vi "AlliGator Refnums Storage.vi"(6 "Get(F)/Set":bool, 7 "AlliGator Refnum List":T1, 8 "Error In":errorcluster, 11 "Data in":variant) -> (0 "Error Out":errorcluster, 3 "Data out":variant)   [LabVIEW 2021, in "AlliGator Globals, Variables & Constants.lvlib"]
doc: "LV2-type global storing refnums to VIs, Tabs and Indicators."
uses:
  AlliGator Globals, Variables & Constants.lvlib
  AlliGator Refnums List.ctl
  GUI/AlliGator Main Window Tabs.ctl
  GUI/AlliGator GUI.lvlib
panel:
  in  "Tab Control":enum32{"Controls", "Indicators", "VIs"}(tab)
  in  "AlliGator Tab Control Refnum":refnum<vi>
  in  "Phasor Plot Display":refnum<vi>
  in  "Decay Fit Parameter Map Display":refnum<vi> caption="Source Image Display"
  in  "Source Image Display":refnum<vi>
  in  "AlliGator Launcher  Refnum":refnum<vi>
  in  "AlliGator Settings Refnum":refnum<vi>
  in  "AlliGator Refnum":refnum<vi>
  # "see the AlliGator License on the block diagram (Ctrl+E or Window:Show Block Diagram)"
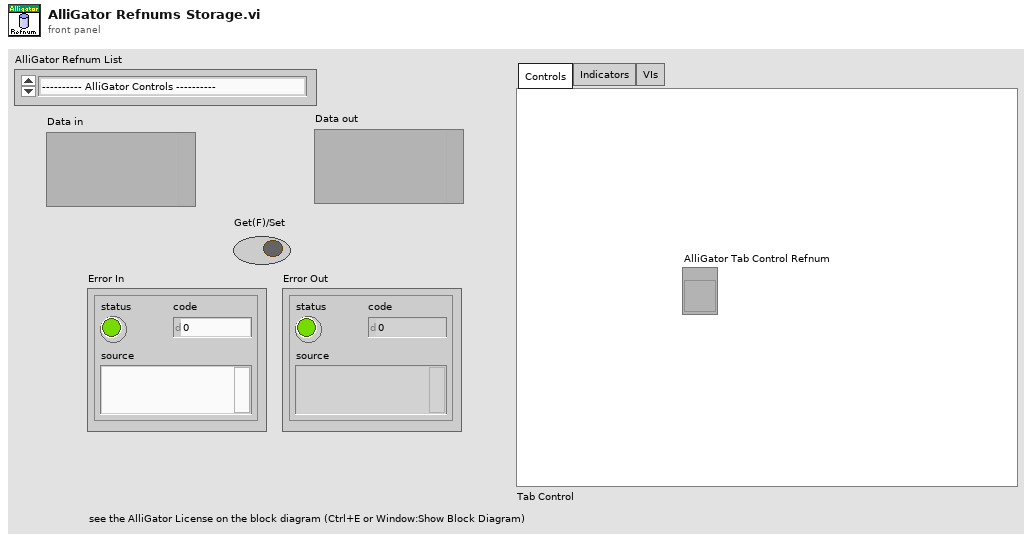
[diagram p1: front panel]
types:
  T1 = typedef "AlliGator Globals, Variables & Constants.lvlib/AlliGator Refnums List.ctl" = enum16{"---------- AlliGator Controls ----------", "AlliGator Tab Control Refnum", "---------- AlliGator Indicators ----------", "Source Image Display Refnum", "Phasor Plot Display Refnum", "Decay Fit Parameter Map Refnum", "---------- AlliGator VIs ----------", "AlliGator Refnum", "AlliGator Settings Refnum", "AlliGator Launcher Refnum"}
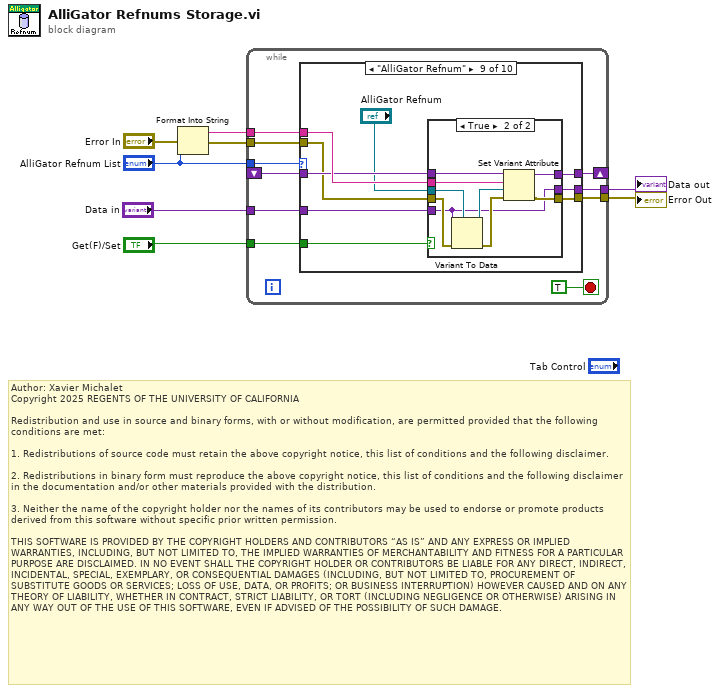
[diagram p0: block diagram]
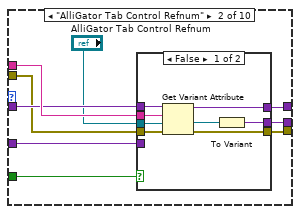
[diagram p3: hidden frame]
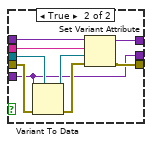
[diagram p4: hidden frame]
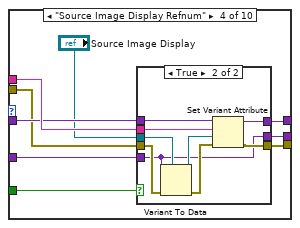
[diagram p6: hidden frame]
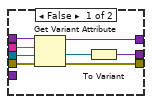
[diagram p7: hidden frame]
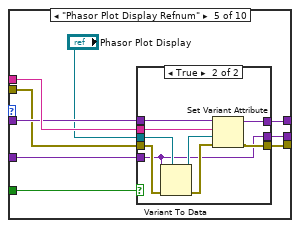
[diagram p8: hidden frame]
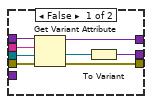
[diagram p9: hidden frame]
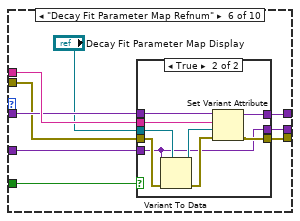
[diagram p10: hidden frame]
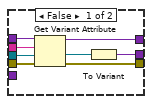
[diagram p11: hidden frame]
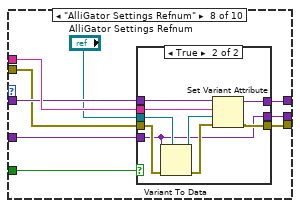
[diagram p13: hidden frame]
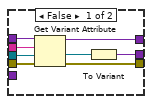
[diagram p14: hidden frame]
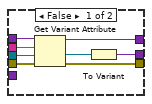
[diagram p15: hidden frame]
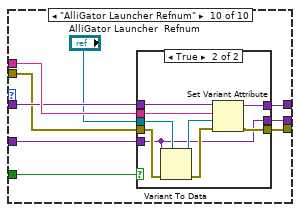
[diagram p16: hidden frame]
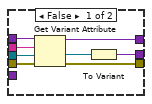
[diagram p17: hidden frame]
diagram:
  # "Author: Xavier Michalet\nCopyright 2025 REGENTS OF THE UNIVERSITY OF CALIFORNIA\n\nRedistribution and use in source and binary forms, with or without modification, are permitted provided that the following conditions are met:\n\n1. Redistributions of source code must retain the above copyright notice, this list of conditions and the following disclaimer.\n\n2. Redistributions in binary form must reproduce the above copyright notice, this list of conditions and the following disclaimer in the documentation and/or other materials provided with the distribution.\n\n3. Neither the name of the copyright holder nor the names of its contributors may be used to endorse or promote products derived from this software without specific prior written permission.\n\nTHIS SOFTWARE IS PROVIDED BY THE COPYRIGHT HOLDERS AND CONTRIBUTORS “AS IS” AND ANY EXPRESS OR IMPLIED WARRANTIES, INCLUDING, BUT NOT LIMITED TO, THE IMPLIED WARRANTIES OF MERCHANTABILITY AND FITNESS FOR A PARTICULAR PURPOSE ARE DISCLAIMED. IN NO EVENT SHALL THE COPYRIGHT HOLDER OR CONTRIBUTORS BE LIABLE FOR ANY DIRECT, INDIRECT, INCIDENTAL, SPECIAL, EXEMPLARY, OR CONSEQUENTIAL DAMAGES (INCLUDING, BUT NOT LIMITED TO, PROCUREMENT OF SUBSTITUTE GOODS OR SERVICES; LOSS OF USE, DATA, OR PROFITS; OR BUSINESS INTERRUPTION) HOWEVER CAUSED AND ON ANY THEORY OF LIABILITY, WHETHER IN CONTRACT, STRICT LIABILITY, OR TORT (INCLUDING NEGLIGENCE OR OTHERWISE) ARISING IN ANY WAY OUT OF THE USE OF THIS SOFTWARE, EVEN IF ADVISED OF THE POSSIBILITY OF SUCH DAMAGE."
  n1 = Format Into String(error in="Error In", "AlliGator Refnum List") -> (resulting string=w7:string, error out=w4:errorcluster)  [unwired: 2 in]
  n2 = while {
    tunnel: "Get(F)/Set" -> [w11]
    tunnel: w7 -> [w17]
    shift-right: [w15] -> _
    shift-left: _ -> [w16]
    tunnel: "Data in" -> [w10]
    tunnel: w4 -> [w14]
    tunnel: [w13] -> w3
    tunnel: [w12] -> w2
    tunnel: "AlliGator Refnum List" -> [w9]
    stop <- TRUE stop-if-true
    n3 = case shown="\"AlliGator Refnum\"" w9 {
      tunnel: w17 -> [_ w30 _ w59 w85 w111 _ w140 w166 w192]
      tunnel: w16 -> [w20 w29 w50 w58 w84 w110 w130 w139 w165 w191]
      tunnel: [w20 w28 w50 w57 w83 w109 w130 w138 w164 w190] -> w15
      tunnel: w14 -> [w21 w27 w48 w56 w82 w108 w131 w137 w163 w189]
      tunnel: [w21 w26 w48 w55 w81 w107 w131 w136 w162 w188] -> w13
      tunnel: [w19 w25 w49 w54 w80 w106 w129 w135 w161 w187] -> w12
      tunnel: w11 -> [_ w24 _ w53 w79 w105 _ w134 w160 w186]
      tunnel: w10 -> [w19 w23 w49 w52 w78 w104 w129 w133 w159 w185]
      frame "---------- AlliGator Controls ----------", Default {
      }
      frame "AlliGator Tab Control Refnum" {
        n4 = case shown="False" w24 {
          tunnel: w29 -> [w38 w47]
          tunnel: w30 -> [w37 w42]
          tunnel: w27 -> [w36 w46]
          tunnel: [w35 w40] -> w26
          tunnel: [w31 w39] -> w25
          tunnel: [w33 w41] -> w28
          tunnel: "AlliGator Tab Control Refnum" -> [w32 w45]
          tunnel: w23 -> [_ w39]
          frame False {
            n5 = Get Variant Attribute(Variant=w38, name=w37, default value (empty Variant)=w32, error in=w36) -> (duplicate Variant=w33:variant, value=w34:refnum<vi>, error out=w35:errorcluster)  [unwired: 1 out]
            n6 = To Variant(anything=w34) -> (Variant=w31:variant)
          }
          frame True {
            n7 = Variant To Data(error in=w46, type=w45, Variant=w39) -> (data=w44:refnum<vi>, error out=w43:errorcluster)
            n8 = Set Variant Attribute(Variant=w47, name=w42, value=w44, error in=w43) -> (Variant out=w41:variant, error out=w40:errorcluster)  [unwired: 1 out]
          }
        }
      }
      frame "---------- AlliGator Indicators ----------" {
      }
      frame "Source Image Display Refnum" {
        n9 = case shown="True" w53 {
          tunnel: w58 -> [w67 w76]
          tunnel: w59 -> [w66 w71]
          tunnel: w56 -> [w65 w75]
          tunnel: [w64 w69] -> w55
          tunnel: [w60 w68] -> w54
          tunnel: [w62 w70] -> w57
          tunnel: "Source Image Display" -> [w61 w74]
          tunnel: w52 -> [_ w68]
          frame False {
            n10 = Get Variant Attribute(Variant=w67, name=w66, default value (empty Variant)=w61, error in=w65) -> (duplicate Variant=w62:variant, value=w63:refnum<vi>, error out=w64:errorcluster)  [unwired: 1 out]
            n11 = To Variant(anything=w63) -> (Variant=w60:variant)
          }
          frame True {
            n12 = Variant To Data(error in=w75, type=w74, Variant=w68) -> (data=w73:refnum<vi>, error out=w72:errorcluster)
            n13 = Set Variant Attribute(Variant=w76, name=w71, value=w73, error in=w72) -> (Variant out=w70:variant, error out=w69:errorcluster)  [unwired: 1 out]
          }
        }
      }
      frame "Phasor Plot Display Refnum" {
        n14 = case shown="True" w79 {
          tunnel: w84 -> [w93 w102]
          tunnel: w85 -> [w92 w97]
          tunnel: w82 -> [w91 w101]
          tunnel: [w90 w95] -> w81
          tunnel: [w86 w94] -> w80
          tunnel: [w88 w96] -> w83
          tunnel: "Phasor Plot Display" -> [w87 w100]
          tunnel: w78 -> [_ w94]
          frame False {
            n15 = Get Variant Attribute(Variant=w93, name=w92, default value (empty Variant)=w87, error in=w91) -> (duplicate Variant=w88:variant, value=w89:refnum<vi>, error out=w90:errorcluster)  [unwired: 1 out]
            n16 = To Variant(anything=w89) -> (Variant=w86:variant)
          }
          frame True {
            n17 = Variant To Data(error in=w101, type=w100, Variant=w94) -> (data=w99:refnum<vi>, error out=w98:errorcluster)
            n18 = Set Variant Attribute(Variant=w102, name=w97, value=w99, error in=w98) -> (Variant out=w96:variant, error out=w95:errorcluster)  [unwired: 1 out]
          }
        }
      }
      frame "Decay Fit Parameter Map Refnum" {
        n19 = case shown="True" w105 {
          tunnel: w110 -> [w119 w128]
          tunnel: w111 -> [w118 w123]
          tunnel: w108 -> [w117 w127]
          tunnel: [w116 w121] -> w107
          tunnel: [w112 w120] -> w106
          tunnel: [w114 w122] -> w109
          tunnel: "Decay Fit Parameter Map Display" -> [w113 w126]
          tunnel: w104 -> [_ w120]
          frame False {
            n20 = Get Variant Attribute(Variant=w119, name=w118, default value (empty Variant)=w113, error in=w117) -> (duplicate Variant=w114:variant, value=w115:refnum<vi>, error out=w116:errorcluster)  [unwired: 1 out]
            n21 = To Variant(anything=w115) -> (Variant=w112:variant)
          }
          frame True {
            n22 = Variant To Data(error in=w127, type=w126, Variant=w120) -> (data=w125:refnum<vi>, error out=w124:errorcluster)
            n23 = Set Variant Attribute(Variant=w128, name=w123, value=w125, error in=w124) -> (Variant out=w122:variant, error out=w121:errorcluster)  [unwired: 1 out]
          }
        }
      }
      frame "---------- AlliGator VIs ----------" {
      }
      frame "AlliGator Settings Refnum" {
        n24 = case shown="True" w134 {
          tunnel: w139 -> [w148 w157]
          tunnel: w140 -> [w147 w152]
          tunnel: w137 -> [w146 w156]
          tunnel: [w145 w150] -> w136
          tunnel: [w141 w149] -> w135
          tunnel: [w143 w151] -> w138
          tunnel: "AlliGator Settings Refnum" -> [w142 w155]
          tunnel: w133 -> [_ w149]
          frame False {
            n25 = Get Variant Attribute(Variant=w148, name=w147, default value (empty Variant)=w142, error in=w146) -> (duplicate Variant=w143:variant, value=w144:refnum<vi>, error out=w145:errorcluster)  [unwired: 1 out]
            n26 = To Variant(anything=w144) -> (Variant=w141:variant)
          }
          frame True {
            n27 = Variant To Data(error in=w156, type=w155, Variant=w149) -> (data=w154:refnum<vi>, error out=w153:errorcluster)
            n28 = Set Variant Attribute(Variant=w157, name=w152, value=w154, error in=w153) -> (Variant out=w151:variant, error out=w150:errorcluster)  [unwired: 1 out]
          }
        }
      }
      frame "AlliGator Refnum" {
        n29 = case shown="True" w160 {
          tunnel: w165 -> [w174 w183]
          tunnel: w166 -> [w173 w178]
          tunnel: w163 -> [w172 w182]
          tunnel: [w171 w176] -> w162
          tunnel: [w167 w175] -> w161
          tunnel: [w169 w177] -> w164
          tunnel: "AlliGator Refnum" -> [w168 w181]
          tunnel: w159 -> [_ w175]
          frame False {
            n30 = Get Variant Attribute(Variant=w174, name=w173, default value (empty Variant)=w168, error in=w172) -> (duplicate Variant=w169:variant, value=w170:refnum<vi>, error out=w171:errorcluster)  [unwired: 1 out]
            n31 = To Variant(anything=w170) -> (Variant=w167:variant)
          }
          frame True {
            n32 = Variant To Data(error in=w182, type=w181, Variant=w175) -> (data=w180:refnum<vi>, error out=w179:errorcluster)
            n33 = Set Variant Attribute(Variant=w183, name=w178, value=w180, error in=w179) -> (Variant out=w177:variant, error out=w176:errorcluster)  [unwired: 1 out]
          }
        }
      }
      frame "AlliGator Launcher Refnum" {
        n34 = case shown="True" w186 {
          tunnel: w191 -> [w200 w209]
          tunnel: w192 -> [w199 w204]
          tunnel: w189 -> [w198 w208]
          tunnel: [w197 w202] -> w188
          tunnel: [w193 w201] -> w187
          tunnel: [w195 w203] -> w190
          tunnel: "AlliGator Launcher  Refnum" -> [w194 w207]
          tunnel: w185 -> [_ w201]
          frame False {
            n35 = Get Variant Attribute(Variant=w200, name=w199, default value (empty Variant)=w194, error in=w198) -> (duplicate Variant=w195:variant, value=w196:refnum<vi>, error out=w197:errorcluster)  [unwired: 1 out]
            n36 = To Variant(anything=w196) -> (Variant=w193:variant)
          }
          frame True {
            n37 = Variant To Data(error in=w208, type=w207, Variant=w201) -> (data=w206:refnum<vi>, error out=w205:errorcluster)
            n38 = Set Variant Attribute(Variant=w209, name=w204, value=w206, error in=w205) -> (Variant out=w203:variant, error out=w202:errorcluster)  [unwired: 1 out]
          }
        }
      }
    }
  }
  "Data out" <- w2
  "Error Out" <- w3
